vi "Saturation Return or End Sequence.vi"(9 "error in (no error)":errorcluster, 10 "return position":dbl, 11 ".NET Refnum in":refnum<k24>) -> (2 "error out":errorcluster, 3 "reference out":refnum<k24>)   [LabVIEW 2023]
uses:
  C:/Users/nanometa/Documents/TCSPC_Git_Repo/Source/ThorLabs.MotionControl.KCube.DCServoCLI.dll
  ThorLabs.MotionControl.KCube.DCServoCLI.dll
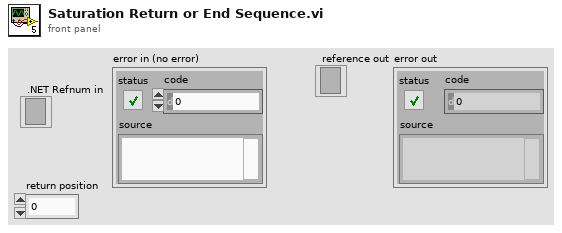
[diagram p1: front panel]
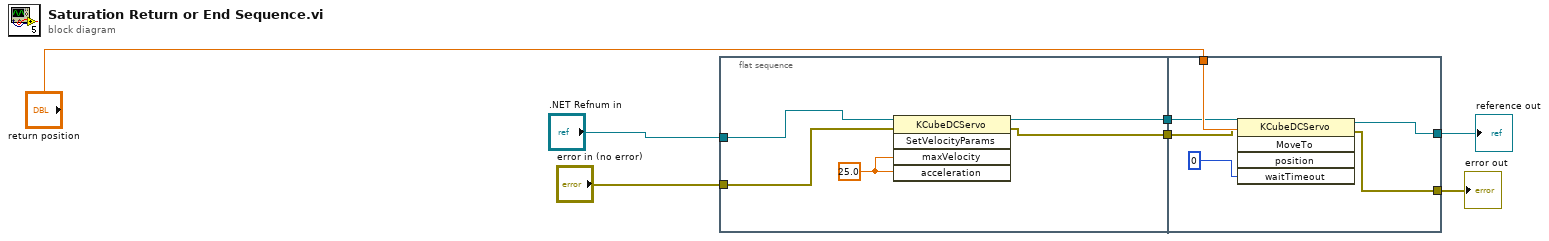
[diagram p0: block diagram]
diagram:
  n1 = flat-sequence {
    tunnel: ".NET Refnum in" -> [w11]
    tunnel: [w10] -> w5
    tunnel: [w9] -> w3
    tunnel: "error in (no error)" -> [w8]
    tunnel: "return position" -> [w17]
    tunnel: w5 -> [w16]
    tunnel: [w15] -> w4
    tunnel: w3 -> [w14]
    tunnel: [w13] -> w2
    frame #0 {
      w12 = 25.0 ("acceleration")
      n2 = invoke class="KCubeDCServo" method="SetVelocityParams"(reference=w11, error in=w8, "maxVelocity"=w12, "acceleration"=w12) -> (reference out=w10:refnum<k24>, error out=w9:errorcluster)  [unwired: 1 in, 3 out]
    }
    frame #1 {
      n3 = invoke class="KCubeDCServo" method="MoveTo"(reference=w16, error in=w14, "position"=w17, "waitTimeout"=0) -> (reference out=w15:refnum<k24>, error out=w13:errorcluster)  [unwired: 1 in, 3 out]
    }
  }
  "reference out" <- w4
  "error out" <- w2
